vi "_Destroy.vi"(8 "error in (no error)":errorcluster, 11 "Scan Driver in":refnum<class "Scan Driver.lvclass">) -> (0 "error out":errorcluster)   [LabVIEW 2009, in "Scan Driver.lvclass"]
uses:
  Scan Driver.lvclass
  Scan Driver.lvclass/Scan Driver.ctl
  Scanners/Scanner/Scanner.lvclass
  Readers/Reader/Reader.lvclass
  Instruments/Utility Classes/Readable/Readable.lvclass
  Instruments/Utility Classes/Scannable/Scannable.lvclass
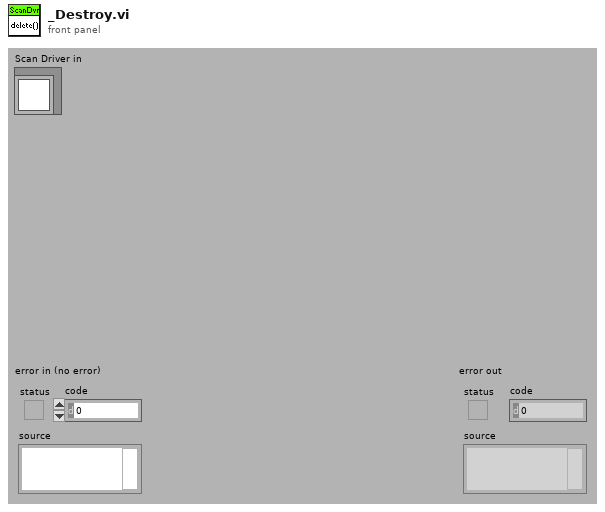
[diagram p1: front panel]
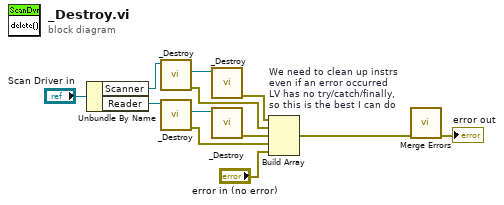
[diagram p0: block diagram]
diagram:
  n1 = Unbundle By Name("Scan Driver in") -> ("Scanner"=w11:refnum<class "Scanner.lvclass">, "Reader"=w9:refnum<class "Reader.lvclass">)
  n2 = call-dynamic "_Destroy.vi"("Scanner in"=w11) -> ("error out"=w6:errorcluster, "finalized Scannable"=w10:refnum<class "Scannable.lvclass">)  [unwired: 1 in, 8 out]
  n3 = call-dynamic "_Destroy.vi"("Reader in"=w9) -> ("error out"=w4:errorcluster, "Finalized Readable"=w8:refnum<class "Readable.lvclass">)  [unwired: 1 in, 8 out]
  n4 = call-dynamic "_Destroy.vi"("Instrument in"=w10) -> ("error out"=w7:errorcluster)  [unwired: 1 in, 9 out]
  n5 = call-dynamic "_Destroy.vi"("Instrument in"=w8) -> ("error out"=w5:errorcluster)  [unwired: 1 in, 9 out]
  n6 = Build Array "We need to clean up instrs\neven if an error occurred\nLV has no try/catch/finally,\nso this is the best I can do"(w7, w6, w5, w4, "error in (no error)") -> (w2:errorcluster[])
  n7 = call <vilib>:"Merge Errors.vi"("error array in"=w2) -> ("error out"=→"error out":errorcluster)  [unwired: 3 in, 3 out]
